vi "Initialize.vi"(7 "VI Ref":variant, 8 "error in (no error)":errorcluster, 9 "Wizard Interface":T1, 10 "MetaDataObj in":refnum<class "MetaDataObj.lvclass">, 11 "BaseSpecPage in":refnum<class "BaseSpecPage.lvclass">) -> (0 "error out":errorcluster, 3 "BaseSpecPage out":refnum<class "BaseSpecPage.lvclass">)   [LabVIEW 2016, in "BaseSpecPage.lvclass"]
uses:
  <resource>/dialog/NewProjectWizard/SpecPage/Base/BaseSpecPage.lvclass
  <resource>/dialog/NewProjectWizard/MetaDataObj/MetaDataObj.lvclass
  <resource>/dialog/NewProjectWizard/Spec Page Interface.ctl
  <resource>/dialog/NewProjectWizard/SpecPage/Base/BaseSpecPage.lvclass/BaseSpecPage.ctl
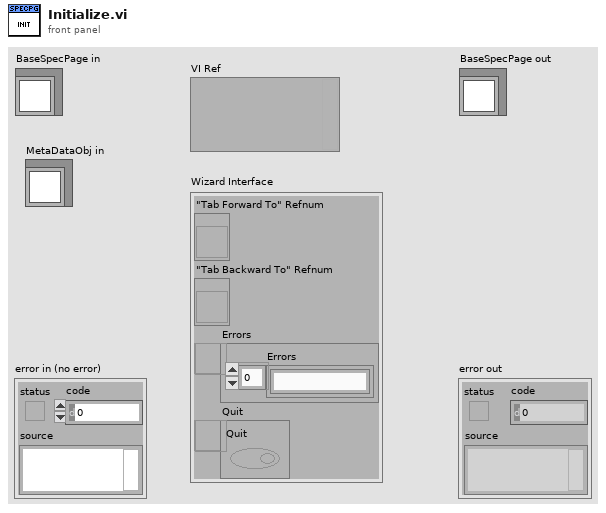
[diagram p1: front panel]
types:
  T1 = typedef "Spec Page Interface.ctl" = cluster{"\"Tab Forward To\" Refnum":refnum<vi>, "\"Tab Backward To\" Refnum":refnum<vi>, "Errors":refnum<user-event>, "Quit":refnum<user-event>}
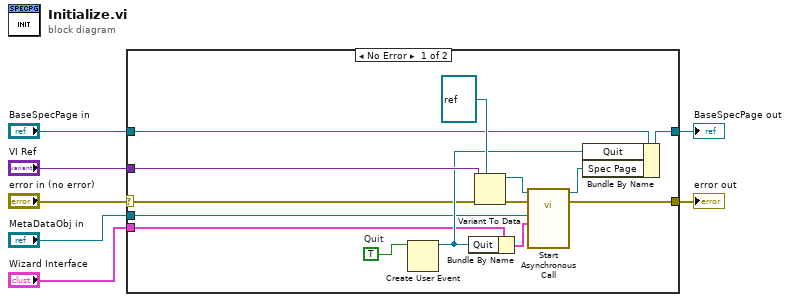
[diagram p0: block diagram]
diagram:
  n1 = case shown="No Error" "error in (no error)" {
    selector: "error in (no error)" -> [w8 w23]
    tunnel: [w9 w23] -> w6
    tunnel: [w16 w22] -> w4
    tunnel: "BaseSpecPage in" -> [w17 w22]
    tunnel: "VI Ref" -> [w18 _]
    tunnel: "MetaDataObj in" -> [w12 _]
    tunnel: "Wizard Interface" -> [w11 _]
    frame No Error {
      w21 = TRUE  # Quit
      n2 = Create User Event(user event datatype=w21) -> (user event=w15:refnum<user-event>)  [unwired: 1 in, 1 out]
      n3 = Bundle By Name(cluster=w11, "Quit"=w15) -> (w13:T1)
      n4 = Variant To Data(error in=w8, type=refnum<vi> refnum ("reference"), Variant=w18) -> (data=w19:refnum<vi>, error out=w10:errorcluster)
      n5 = call-by-ref "Start Asynchronous Call"(reference=w19, error in=w10, "Spec Page Interface"=w13, "MetaDataObj in"=w12) -> (reference out=w14:refnum<vi>, error out=w9:errorcluster)  [unwired: 9 in, 1 out]
      n6 = Bundle By Name(cluster=w17, "Quit"=w15, "Spec Page"=w14) -> (w16:refnum<class "BaseSpecPage.lvclass">)
    }
    frame Error {
    }
  }
  "error out" <- w6
  "BaseSpecPage out" <- w4
